vi "get channels.vi"(11 "UI Reference configuration in":refnum<class "UI Reference configuration.lvclass">) -> (2 "channels":refnum<class "TBM channel.lvclass">[](array[class]), 3 "UI Reference configuration out":refnum<class "UI Reference configuration.lvclass">)   [LabVIEW 2013, in "UI Reference configuration.lvclass"]
uses:
  UI Reference configuration.lvclass
  <vilib>/NI/Tag Bus Module Framework/channel/TBM channel.lvclass
  UI Reference configuration.lvclass/UI Reference configuration.ctl
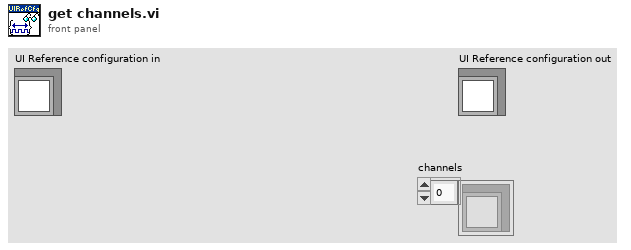
[diagram p1: front panel]
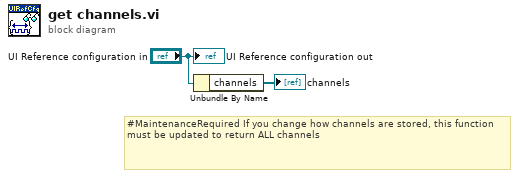
[diagram p0: block diagram]
diagram:
  # "#MaintenanceRequired If you change how channels are stored, this function must be updated to return ALL channels"
  n1 = Unbundle By Name("UI Reference configuration in") -> ("channels"=→"channels":refnum<class "TBM channel.lvclass">[])
  "UI Reference configuration out" <- "UI Reference configuration in"
